vi "RSZVB Set Linearity Deviation Constant.vi"(8 "error in (no error)":errorcluster {"code" format="%.0x"}, 9 "Constant (0.0 dB)":dbl format="%^.3e", 10 "Channel (1)":i32=1, 11 "VISA session":refnum<visa-resource-name>) -> (0 "error out":errorcluster {"code" format="%.0x"}, 3 "dup VISA session":refnum<visa-resource-name>)   [LabVIEW 2011]
doc: "This VI defines the constant value for the linearity deviation calculation.\n\nRemote-control command(s):\nCALCulate<Chn>:LDEViation:CONStant"
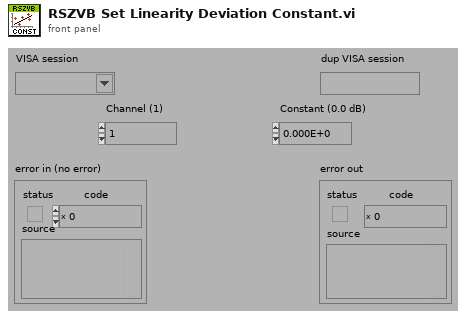
[diagram p1: front panel]
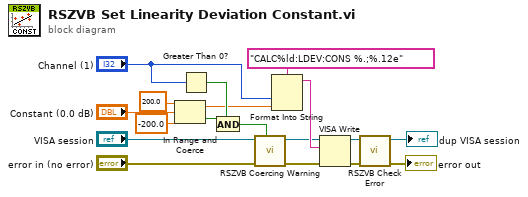
[diagram p0: block diagram]
diagram:
  n1 = In Range and Coerce(upper limit=200.0, x="Constant (0.0 dB)", lower limit=-200.0) -> (coerced(x)=w7:dbl, In Range?=w10:bool)
  n2 = Greater Than 0?(x="Channel (1)") -> (x > 0?=w9:bool)
  n3 = And(x=w9, y=w10) -> (x .and. y?=w11:bool)
  n4 = call "RSZVB Coercing Warning.vi"("In Range?"=w11, "error in (no error)"="error in (no error)", "VISA session"="VISA session") -> ("error out"=w5:errorcluster, "dup VISA session"=w13:refnum<visa-resource-name>)  [unwired: 7 in]
  n5 = Format Into String(format string="CALC%ld:LDEV:CONS %.;%.12e", "Channel (1)", w7) -> (resulting string=w17:string)  [unwired: 2 in, 1 out]
  n6 = VISA Write(VISA resource name=w13, write buffer=w17, error in (no error)=w5) -> (VISA resource name out=w4:refnum<visa-resource-name>, error out=w3:errorcluster)  [unwired: 1 out]
  n7 = call "RSZVB Check Error.vi"("error in (no error)"=w3, "VISA session"=w4) -> ("error out"=→"error out":errorcluster, "dup VISA session"=→"dup VISA session":refnum<visa-resource-name>)  [unwired: 8 in]
